vi "SUB_COM_NoErrRead_count.vi"(8 "read count":i32, 9 "VISA resource name":refnum<visa-resource-name>) -> (1 "concatenated string":string, 3 "VISA resource name out":refnum<visa-resource-name>)   [LabVIEW 2011]
panel:
  out "Numeric":i32
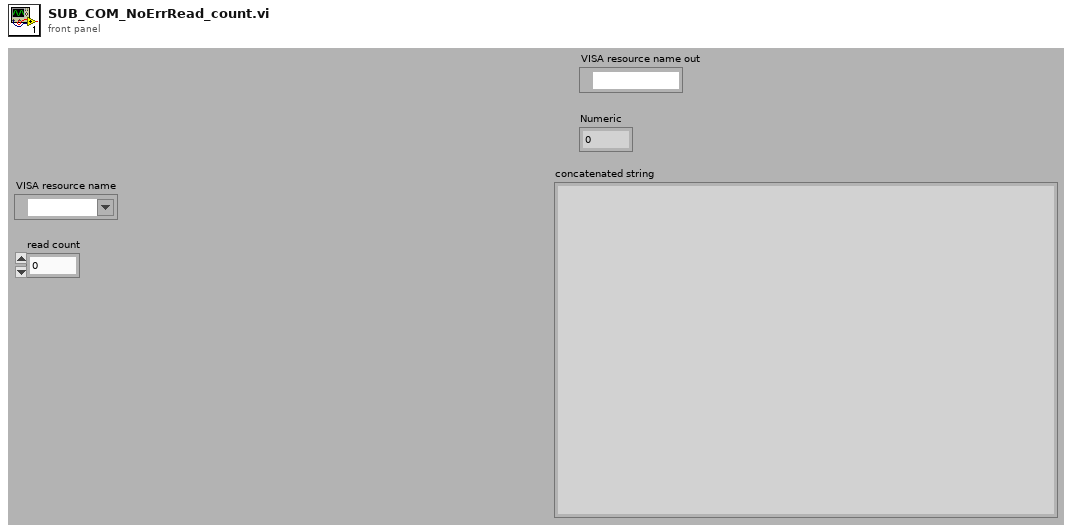
[diagram p1: front panel]
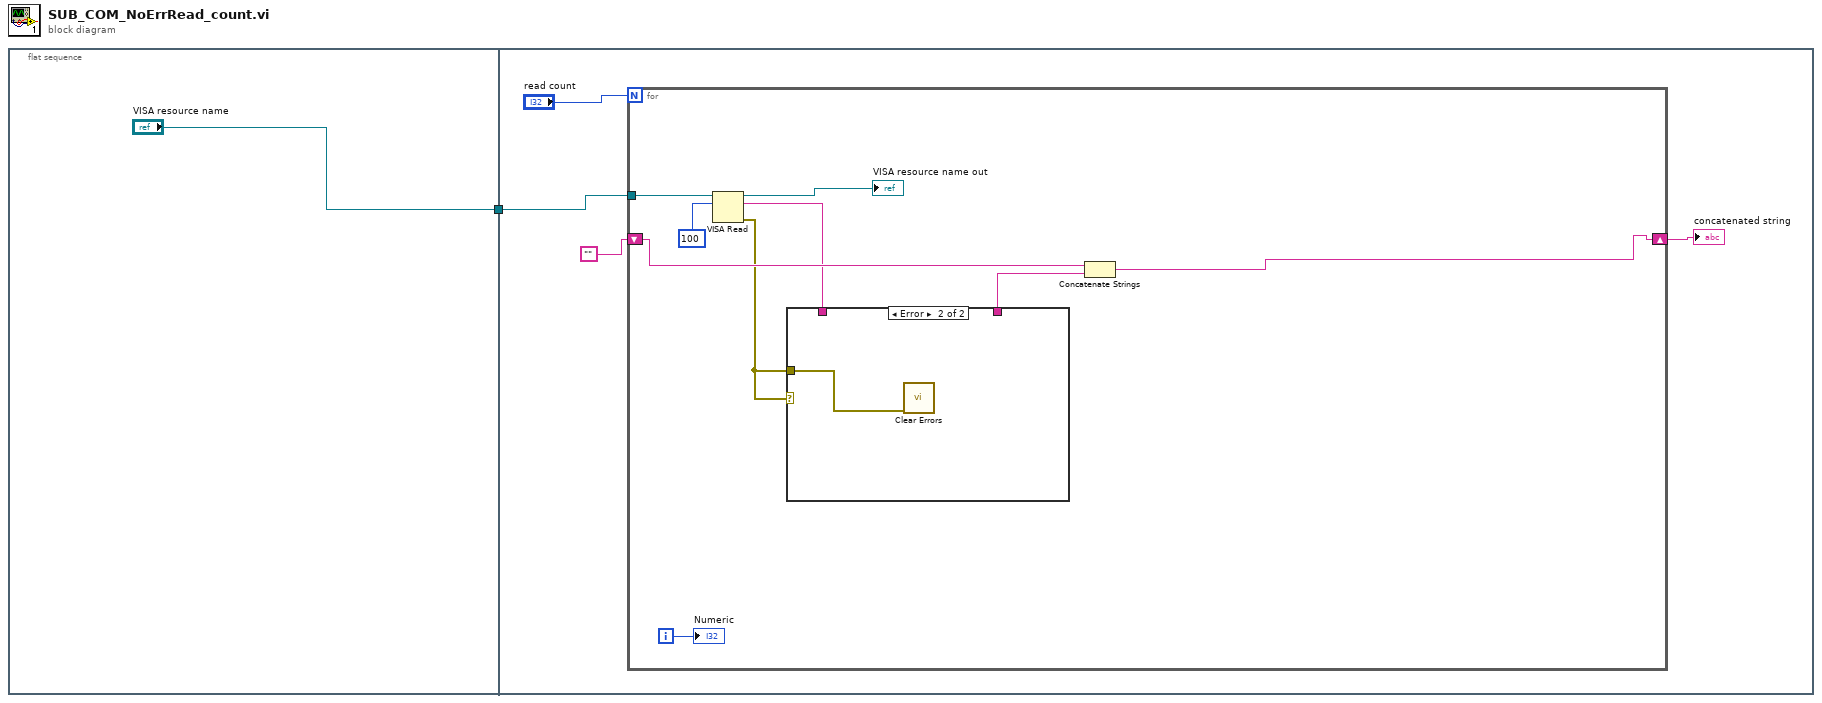
[diagram p0: block diagram]
diagram:
  n1 = flat-sequence {
    tunnel: ["VISA resource name"] -> w1
    tunnel: w1 -> [w5]
    frame #0 {
    }
    frame #1 {
      n2 = for {
        N: "read count" -> [_]
        shift-right: [w14] -> w4
        shift-left: "" -> [w15]
        tunnel: w5 -> [w11]
        i -> [w13]
        n3 = VISA Read(VISA resource name=w11, byte count=u32 100 ("bytes to read")) -> (VISA resource name out=→"VISA resource name out":refnum<visa-resource-name>, read buffer=w8:string, error out=w7:errorcluster)  [unwired: 1 in, 1 out]
        n4 = case shown="Error" w7 {
          tunnel: [w16 _] -> w9
          tunnel: w8 -> [w16 _]
          tunnel: w7 -> [_ w17]
          frame No Error {
          }
          frame Error {
            n5 = call <vilib>:"Clear Errors.vi"("error in (no error)"=w17) -> ()  [unwired: 6 in, 1 out]
          }
        }
        n6 = Concatenate Strings(w15, w9) -> (w14:string)
        "Numeric" <- w13
      }
      "concatenated string" <- w4
    }
  }
